vi "Initialize.vi"(8 "error in (no error)":errorcluster, 10 "Array of Hardware":refnum<class "Hardware.lvclass">[](array[class]), 11 "VacuumLines in":refnum<class "VacuumLines.lvclass">) -> (0 "error out":errorcluster, 2 "error in labels?":bool, 3 "VacuumLines out":refnum<class "VacuumLines.lvclass">)   [LabVIEW 2016, in "Hardware.lvlib" / "VacuumLine.lvlib" / "VacuumLines.lvclass"]
uses:
  <userlib>/Common Components/Hardware/Abstract System/VacuumLine/VacuumLines/VacuumLines.lvclass
  <userlib>/Common Components/Hardware/Abstract Hardware/Hardware.lvclass
  <userlib>/Common Components/Hardware/Abstract Hardware/Hardware.lvclass/Hardware.ctl
  <userlib>/Common Components/Hardware/Motor/Motor/Motor.lvclass
  <userlib>/Common Components/Hardware/Displacement Sensor/DispSnsr/DispSnsr.lvclass
  <userlib>/Common Components/Hardware/LogicIO/LogicIO/LogicIO.lvclass
  <userlib>/Common Components/Hardware/GaugeController/GaugeController/GaugeController.lvclass
  <userlib>/Common Components/Hardware/Thermometer/Thermometer.lvclass
  <userlib>/Common Components/Hardware/Abstract System/VacuumLine/VacuumLine/VacuumLine.lvclass
  <userlib>/Common Components/Hardware/Abstract System/VacuumLine/VacuumLine/VacuumLine.lvclass/VacuumLine.ctl
  <userlib>/Common Components/Hardware/Abstract System/VacuumLine/VacuumLines/VacuumLines.lvclass/VacuumLines.ctl
  <userlib>/Common Components/Hardware/Abstract Hardware/Read Label.vi
  <userlib>/Common Components/Hardware/Abstract System/VacuumLine/VacuumLine/Write Motor Obj.vi
  <userlib>/Common Components/Hardware/Abstract System/VacuumLine/VacuumLine/Write DispSnsr Obj.vi
  <userlib>/Common Components/Hardware/Abstract System/VacuumLine/VacuumLine/Write Label.vi
  <userlib>/_OpenG.lib/array/array.llb/Sort 1D Array (String)__ogtk.vi
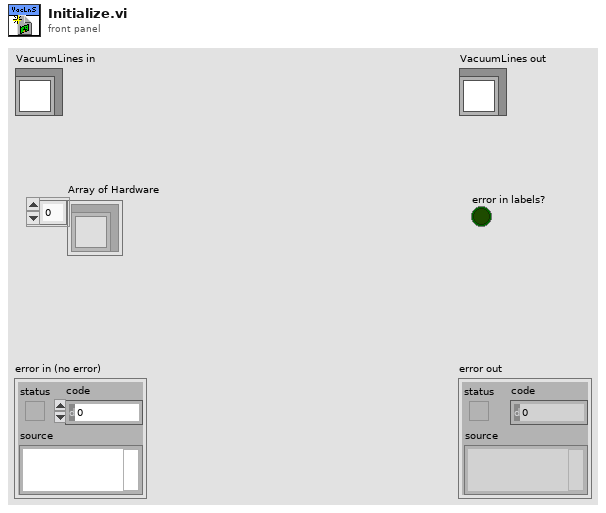
[diagram p1: front panel]
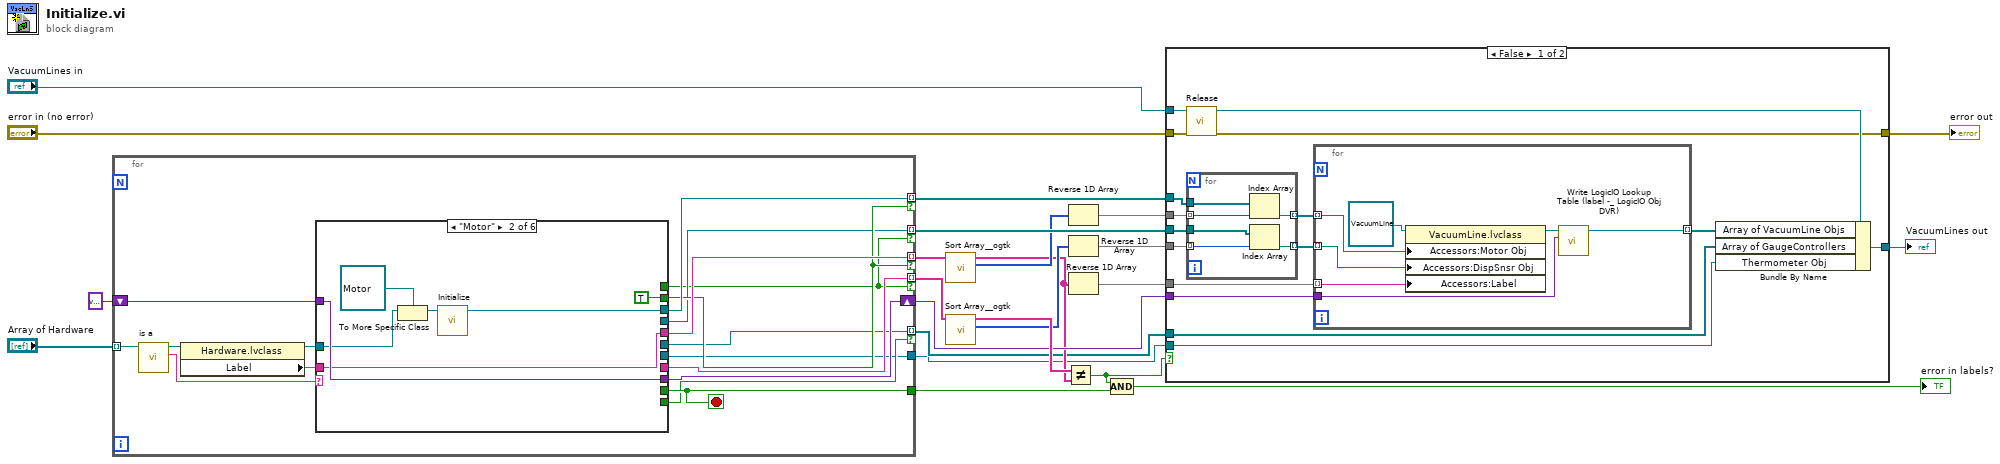
[diagram p0: block diagram]
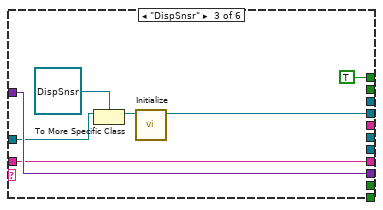
[diagram p4: hidden frame]
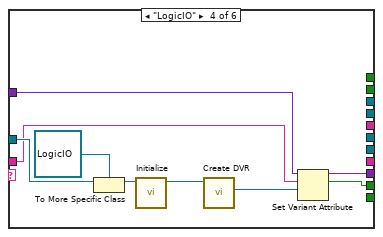
[diagram p5: hidden frame]
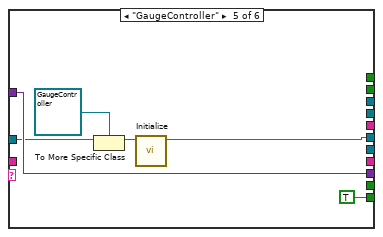
[diagram p6: hidden frame]
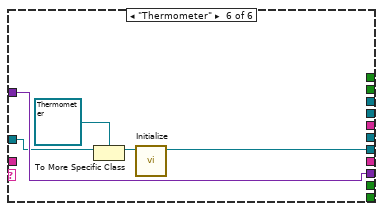
[diagram p7: hidden frame]
diagram:
  n1 = for {
    tunnel: "Array of Hardware" -> [w37] mode=indexing
    shift-right: [w39] -> w11
    shift-left: variant -> [w40]
    tunnel: [w38] -> w21
    tunnel: [w32] -> w20 mode=indexing if=w30
    tunnel: [w31] -> w13 mode=indexing if=w30
    tunnel: [w29] -> w19 mode=indexing if=w27
    tunnel: [w28] -> w15 mode=indexing if=w27
    tunnel: [w26] -> w6 mode=indexing if=w25
    tunnel: [w24] -> w2
    stop <- w38 stop-if-true
    n2 = call-dynamic "is a.vi"("Hardware in"=w37) -> ("is a"=w35:string, "Hardware out"=w36:refnum<class "Hardware.lvclass">)  [unwired: 8 in, 1 out]
    n3 = property class="Hardware.lvclass"(reference=w36) -> (reference out=w34:refnum<class "Hardware.lvclass">, "Label"=w33:string)  [unwired: 1 in, 1 out]
    n4 = case shown="\"Motor\"" w35 {
      tunnel: w40 -> [w41 w48 w55 w64 w70 w75]
      tunnel: [w41 w48 w55 w63 w70 w75] -> w39
      tunnel: [_ _ _ w62 _ _] -> w38
      tunnel: w34 -> [_ w44 w51 w61 w67 w74]
      tunnel: [_ TRUE _ _ _ _] -> w30
      tunnel: w33 -> [_ w46 w54 w59 _ _]
      tunnel: [_ w46 _ _ _ _] -> w32
      tunnel: [_ w42 _ _ _ _] -> w31
      tunnel: [_ _ w54 _ _ _] -> w29
      tunnel: [_ _ TRUE _ _ _] -> w27
      tunnel: [_ _ w49 _ _ _] -> w28
      tunnel: [_ _ _ _ w66 _] -> w26
      tunnel: [_ _ _ _ TRUE _] -> w25
      tunnel: [_ _ _ _ _ w71] -> w24
      frame Default {
      }
      frame "Motor" {
        n5 = To More Specific Class(target class=refnum<class "Motor.lvclass"> refnum ("Hardware.lvlib:Motor.lvlib:Motor.lvclass"), reference=w44) -> (specific class reference=w43:refnum<class "Motor.lvclass">)  [unwired: 1 in, 1 out]
        n6 = call-dynamic "Initialize.vi"("CCD in"=w43) -> ("CCD out"=w42:refnum<class "Motor.lvclass">)  [unwired: 9 in, 1 out]
      }
      frame "DispSnsr" {
        n7 = To More Specific Class(target class=refnum<class "DispSnsr.lvclass"> refnum ("Hardware.lvlib:Displacement Sensor.lvlib:DispSnsr.lvclass"), reference=w51) -> (specific class reference=w50:refnum<class "DispSnsr.lvclass">)  [unwired: 1 in, 1 out]
        n8 = call-dynamic "Initialize.vi"("Hardware in"=w50) -> ("Hardware out"=w49:refnum<class "DispSnsr.lvclass">)  [unwired: 9 in, 1 out]
      }
      frame "LogicIO" {
        n9 = To More Specific Class(target class=refnum<class "LogicIO.lvclass"> refnum ("Hardware.lvlib:LogicIO.lvlib:LogicIO.lvclass"), reference=w61) -> (specific class reference=w58:refnum<class "LogicIO.lvclass">)  [unwired: 1 in, 1 out]
        n10 = call-dynamic "Initialize.vi"("LogicIO in"=w58) -> ("LogicIO out"=w57:refnum<class "LogicIO.lvclass">)  [unwired: 9 in, 1 out]
        n11 = call <userlib>:"Create DVR.vi"("LogicIO in"=w57) -> ("data value reference"=w56:refnum<data-value>)  [unwired: 8 in, 2 out]
        n12 = Set Variant Attribute(Variant=w64, name=w59, value=w56) -> (Variant out=w63:variant, replaced=w62:bool)  [unwired: 1 in, 1 out]
      }
      frame "GaugeController" {
        n13 = To More Specific Class(target class=refnum<class "GaugeController.lvclass"> refnum ("Hardware.lvlib:GaugeController.lvlib:GaugeController.lvclass"), reference=w67) -> (specific class reference=w68:refnum<class "GaugeController.lvclass">)  [unwired: 1 in, 1 out]
        n14 = call-dynamic "Initialize.vi"("Hardware in"=w68) -> ("Hardware out"=w66:refnum<class "GaugeController.lvclass">)  [unwired: 9 in, 1 out]
      }
      frame "Thermometer" {
        n15 = To More Specific Class(target class=refnum<class "Thermometer.lvclass"> refnum ("Hardware.lvlib:Thermometer.lvlib:Thermometer.lvclass"), reference=w74) -> (specific class reference=w72:refnum<class "Thermometer.lvclass">)  [unwired: 1 in, 1 out]
        n16 = call-dynamic "Initialize.vi"("Hardware in"=w72) -> ("Hardware out"=w71:refnum<class "Thermometer.lvclass">)  [unwired: 9 in, 1 out]
      }
    }
  }
  n17 = call-poly <userlib>:"Sort Array__ogtk.vi"("Array in"=w20) -> ("Sorted Pointers"=w12:i32[], "Sorted Array out"=w10:string[])  [unwired: 9 in]
  n18 = call-poly <userlib>:"Sort Array__ogtk.vi"("Array in"=w19) -> ("Sorted Pointers"=w14:i32[], "Sorted Array out"=w16:string[])  [unwired: 9 in]
  n19 = Not Equal?(x=w16, y=w10) -> (x != y?=w17:bool)
  n20 = Reverse 1D Array(array=w12) -> (reversed array=w5:i32[])
  n21 = Reverse 1D Array(array=w14) -> (reversed array=w4:i32[])
  n22 = Reverse 1D Array(array=w10) -> (reversed array=w1:string[])
  n23 = Compound Arithmetic op=AND(w17, w21) -> (→"error in labels?":bool)
  n24 = case shown="False" w17 {
    tunnel: w1 -> [w78 _]
    tunnel: w15 -> [w91 _]
    tunnel: w4 -> [w90 _]
    tunnel: w13 -> [w89 _]
    tunnel: w5 -> [w88 _]
    tunnel: w11 -> [w85 _]
    tunnel: "VacuumLines in" -> [w83 w105]
    tunnel: "error in (no error)" -> [w81 w106]
    tunnel: [w80 w106] -> w7
    tunnel: [w79 w105] -> w3
    tunnel: w6 -> [w77 _]
    tunnel: w2 -> [w76 _]
    frame False {
      n25 = call <userlib>:"Release.vi"("error in (no error)"=w81, "VacuumLines in"=w83) -> ("error out"=w80:errorcluster, "VacuumLines out"=w84:refnum<class "VacuumLines.lvclass">)  [unwired: 8 in]
      n26 = for {
        tunnel: w88 -> [w97] mode=indexing
        tunnel: w89 -> [w96]
        tunnel: [w95] -> w86 mode=indexing
        tunnel: w91 -> [w94]
        tunnel: w90 -> [w93] mode=indexing
        tunnel: [w92] -> w87 mode=indexing
        n27 = Index Array(array=w96, index=w97) -> (element=w95:refnum<class "Motor.lvclass">)
        n28 = Index Array(array=w94, index=w93) -> (element=w92:refnum<class "DispSnsr.lvclass">)
      }
      n29 = for {
        tunnel: w78 -> [w98] mode=indexing
        tunnel: w87 -> [w99] mode=indexing
        tunnel: w86 -> [w100] mode=indexing
        tunnel: w85 -> [w103]
        tunnel: [w102] -> w82 mode=indexing
        n30 = property class="VacuumLine.lvclass"(reference=refnum<class "VacuumLine.lvclass"> refnum ("Hardware.lvlib:VacuumLine.lvlib:VacuumLine.lvclass"), "Accessors:Motor Obj"=w100, "Accessors:DispSnsr Obj"=w99, "Accessors:Label"=w98) -> (reference out=w101:refnum<class "VacuumLine.lvclass">)  [unwired: 1 in, 1 out]
        n31 = call <userlib>:"Write LogicIO Lookup Table (label -_ LogicIO Obj DVR).vi"("LogicIO Lookup Table (label -> LogicIO Obj DVR)"=w103, "VacuumLine in"=w101) -> ("VacuumLine out"=w102:refnum<class "VacuumLine.lvclass">)  [unwired: 9 in]
      }
      n32 = Bundle By Name(cluster=w84, "Array of VacuumLine Objs"=w82, "Array of GaugeControllers"=w77, "Thermometer Obj"=w76) -> (w79:refnum<class "VacuumLines.lvclass">)
    }
    frame True {
    }
  }
  "error out" <- w7
  "VacuumLines out" <- w3
